vi "CANopenVM.vi"() -> ()   [LabVIEW 2020]
uses:
  <vilib>/Platform/TimedLoop/XDataNode/timing_clust.ctl
  <vilib>/Platform/TimedLoop/XDataNode/nitl_modes.ctl
  <vilib>/Platform/TimedLoop/XDataNode/wakeup.ctl
  <vilib>/CANopenLib/CANOPEN.llb/CANopen Interface Create.vi
  <vilib>/CANopenLib/CANOPEN.llb/CANopen SDO Create.vi
  <vilib>/CANopenLib/CANOPEN.llb/CANopen SDO Write [I16].vi
  <vilib>/CANopenLib/CANOPEN.llb/CANopen SDO Close.vi
  <vilib>/CANopenLib/CANOPEN.llb/CANopen SYNC Create.vi
  <vilib>/CANopenLib/CANOPEN.llb/CANopen RPDO Create.vi
  <vilib>/CANopenLib/CANOPEN.llb/CANopen TPDO Create.vi
  <vilib>/CANopenLib/CANOPEN.llb/CANopen SYNC Start.vi
  <vilib>/CANopenLib/CANOPEN.llb/CANopen RPDO Start.vi
  <vilib>/CANopenLib/CANOPEN.llb/CANopen TPDO Start.vi
  <vilib>/CANopenLib/CANOPEN.llb/CANopen Fetch from Data [I32].vi
  <vilib>/CANopenLib/CANOPEN.llb/CANopen SYNC Close.vi
  <vilib>/CANopenLib/CANOPEN.llb/CANopen RPDO Close.vi
  <vilib>/CANopenLib/CANOPEN.llb/CANopen TPDO Close.vi
  <vilib>/CANopenLib/CANOPEN.llb/CANopen Interface Close.vi
  <vilib>/Platform/TimedLoop/XDataNode/XDataNode.xnode
  <vilib>/Platform/TimedLoop/XDataNode/XDNodeRunTimeDep.lvlib
panel:
  in  "数值":i16
  in  "RPDO data":u8[](array[numeric])=[0, 0, 0, 0, 0, 0, 0, 0]
  out "实际速度":i32
  in  "Set Target Vilocity":i16
  in  "stop":bool
  out "timestamp":timestamp=timestamp(11705972400 s since 1904-01-01)
  out "channel data read":i32
  out "CANopen raw data read":u8[](array[numeric])
  in  "buffer size (0)":u16=10
  in  "TPDO channel read":u8(ring)=1 items=["PDO 1", "PDO 2", "PDO 3", "PDO 4"]
  in  "RPDO channel write":u8(ring)=1 items=["PDO 1", "PDO 2", "PDO 3", "PDO 4"]
  in  "period (ms)":i64=10
  out "completion code 2":u32
  out "completion code 1":u32
  in  "batch SDO name":string="NiMotion_VM"
  in  "node-ID":u8=1 min=1 max=127 step=1
  in  "baud rate":u32(ring) items=["1 Mbit/s"=0, "800 kbit/s"=1, "500 kbit/s"=2, "250 kbit/s"=3, "125 kbit/s"=4, "50 kbit/s"=6, "20 kbit/s"=7, "10 kbit/s"=8]
  in  "CANopen interface":u32(ring) items=["CANopen01", "CANopen02", "CANopen03", "CANopen04", "CANopen05", "CANopen06", "CANopen07", "CANopen08", "CANopen09", "CANopen10", "CANopen11", "CANopen12", "CANopen13", "CANopen14", "CANopen15", "CANopen16", "CANopen17", "CANopen18", "CANopen19", "CANopen20", "CANopen21", "CANopen22", "CANopen23", "CANopen24", "CANopen25", "CANopen26", "CANopen27", "CANopen28", "CANopen29", "CANopen30", "CANopen31", "CANopen32"]
  # "601 2B 02 20 01 00 00 00 00"
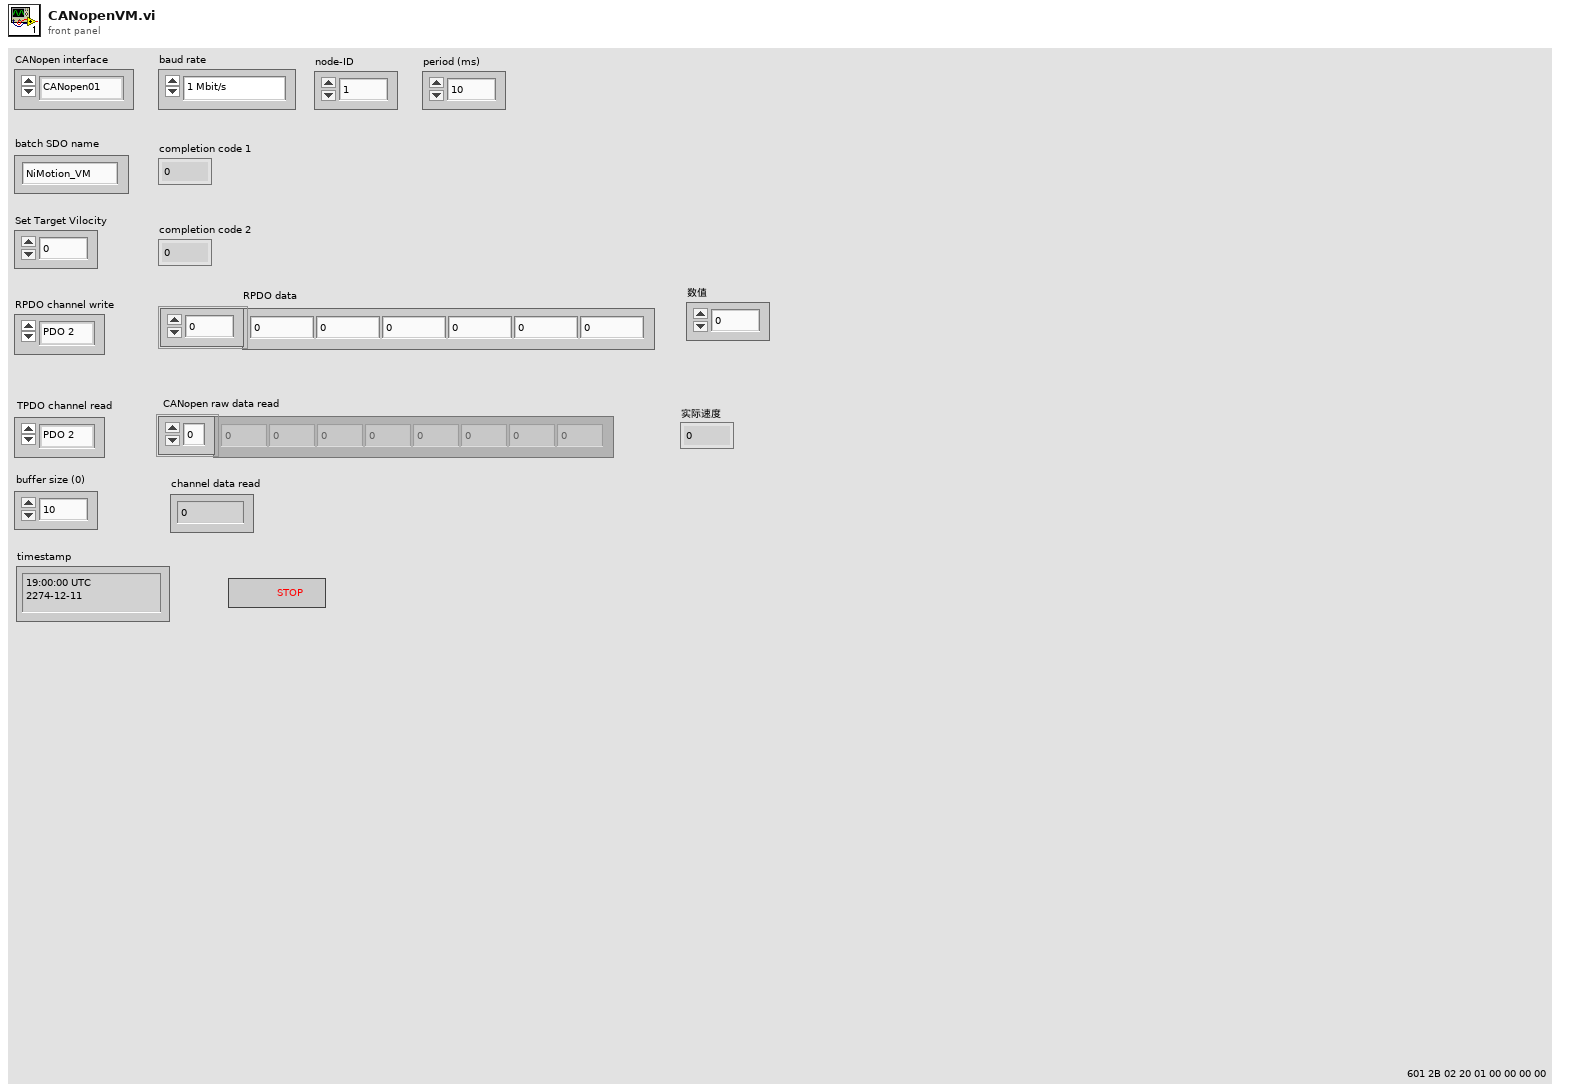
[diagram p1: front panel]
types:
  T1 = typedef "XDNodeRunTimeDep.lvlib/timing_clust.ctl" = cluster{"Expected End [f-1]":u64, "Actual End [f-1]":u64, "Finished Late? [f-1]":bool, "Expected End [i-1]":u64, "Actual End [i-1]":u64, "Finished Late? [i-1]":bool, "Expected Start [i]":u64, "Actual Start [i]":u64, "Expected Start [f]":u64, "Actual Start [f]":u64, "Source Name":string, "Structure Name":string, "Period":i64, "Deadline":i64, "Offset":i64, "Start":i64, "Priority":i32, "Timeout":i32, "Mode":T2, "Wakeup Reason":T3, "Error":errorcluster, "Source Type":string, "Secondary Source Type":string, "Global End Time":u64, "Global Start Time":u64, "Frame Duration":u64, "Iteration Duration":u64, "Assigned CPU":i32, "I/O Scan Engine Mode":u32}
  T2 = typedef "XDNodeRunTimeDep.lvlib/nitl_modes.ctl" = enum32{"No Change", "Process missed periods, maintain original phase", "Discard missed periods, maintain original phase", "Process missed periods, ignore original phase", "Discard missed periods, ignore original phase"}
  T3 = typedef "XDNodeRunTimeDep.lvlib/wakeup.ctl" = enum32{"Normal", "Aborted", "Asynchronous wakeup", "Timing source error", "Timed loop error", "Timeout"}
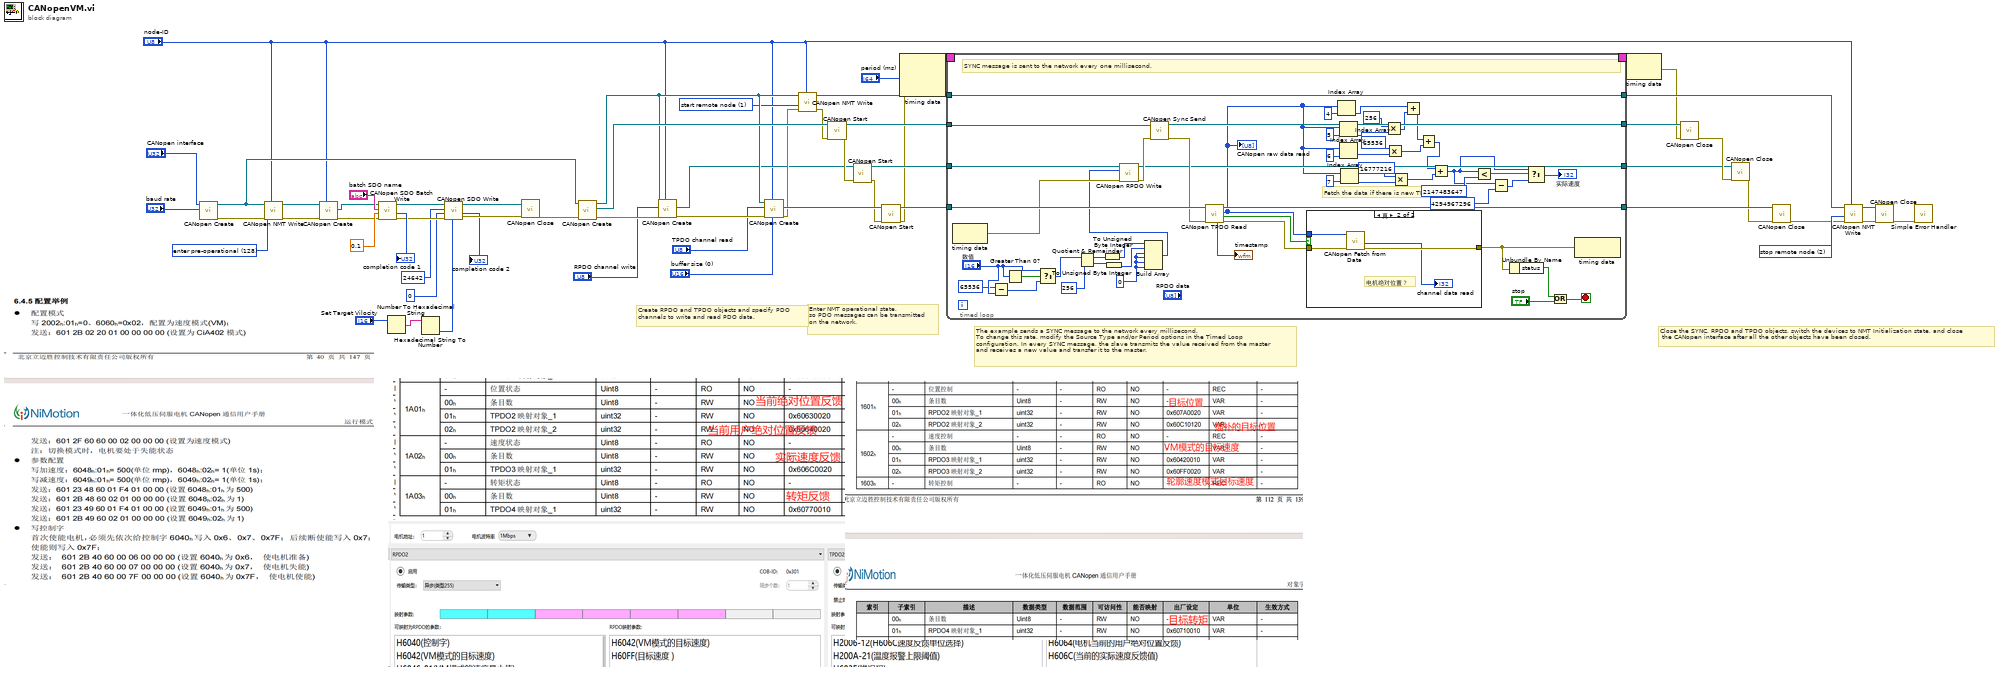
[diagram p0: block diagram]
diagram:
  w20 = u16 2 items=["start remote node"=1, "stop remote node"=2, "enter pre-operational"=128, "reset node"=129, "reset communication"=130] ("command")
  w35 = u16 1 items=["start remote node"=1, "stop remote node"=2, "enter pre-operational"=128, "reset node"=129, "reset communication"=130] ("command")
  w53 = u16 128 items=["start remote node"=1, "stop remote node"=2, "enter pre-operational"=128, "reset node"=129, "reset communication"=130] ("command")
  # "Close the SYNC, RPDO and TPDO objects, switch the devices to NMT Initialization state, and close\n the CANopen interface after all the other objects have been closed."
  # "The example sends a SYNC message to the network every millisecond.\nTo change this rate, modify the Source Type and/or Period options in the Timed Loop\nconfiguration. In every SYNC message, the slave transmits the value received from the master\nand receives a new value and transfer it to the master."
  # "Enter NMT operational state,\nso PDO messages can be transmitted\non the network."
  # "Create RPDO and TPDO objects and specify PDO \nchannels to write and read PDO data."
  n1 = call-poly <vilib>:"CANopen Create.vi"("baud rate"="baud rate", "interface name"="CANopen interface") -> ("error out"=w54:errorcluster, "interface object out"=w26:refnum<k20>)  [unwired: 8 in]
  n2 = call <vilib>:"CANopen NMT Write.vi"("node-ID (0)"="node-ID", "error in (no error)"=w54, "command"=w53, "interface object in"=w26) -> ("error out"=w57:errorcluster, "interface object out"=w58:refnum<k20>)  [unwired: 6 in]
  n3 = call-poly <vilib>:"CANopen Create.vi"("node-ID"="node-ID", "error in (no error)"=w57, "interface object in"=w58) -> ("error out"=w44:errorcluster, "SDO object out"=w50:refnum<k20>)  [unwired: 6 in, 1 out]
  n4 = call <vilib>:"CANopen SDO Batch Write.vi"("error in (no error)"=w44, "timeout (1s)"=0.1 ("timeout (0s)"), "batch SDO name"="batch SDO name", "SDO object in"=w50) -> ("error out"=w45:errorcluster, "completion code"=→"completion code 1":u32, "SDO object out"=w48:refnum<k20>)  [unwired: 5 in]
  n5 = Number To Hexadecimal String(2:"Set Target Vilocity") -> (0:w3:string)  [unwired: 1 in]
  n6 = Hexadecimal String To Number(string=w3) -> (number=w1:u32)  [unwired: 2 in, 1 out]
  n7 = call-poly <vilib>:"CANopen SDO Write.vi"("I16 data"=w1, "error in (no error)"=w45, "object sub-index (0)"=u8 0, "object index"=u16 24642, "SDO object in"=w48) -> ("error out"=w46:errorcluster, "completion code"=→"completion code 2":u32, "SDO object out"=w47:refnum<k20>)  [unwired: 4 in]
  n8 = call-poly <vilib>:"CANopen Close.vi"("error in (no error)"=w46, "SDO object in"=w47) -> ("error out"=w25:errorcluster)  [unwired: 9 in]
  n9 = call-poly <vilib>:"CANopen Create.vi"("error in (no error)"=w25, "interface object in"=w26) -> ("error out"=w38:errorcluster, "SYNC object out"=w37:refnum<k20>, "interface object out"=w36:refnum<k20>)  [unwired: 7 in]
  n10 = call-poly <vilib>:"CANopen Create.vi"("node-ID"="node-ID", "error in (no error)"=w38, "PDO channel"="RPDO channel write", "interface object in"=w36) -> ("error out"=w30:errorcluster, "RPDO object out"=w29:refnum<k20>)  [unwired: 5 in, 1 out]
  n11 = call-poly <vilib>:"CANopen Create.vi"("buffer size (0)"="buffer size (0)", "node-ID"="node-ID", "error in (no error)"=w30, "PDO channel"="TPDO channel read", "interface object in"=w36) -> ("error out"=w34:errorcluster, "TPDO object out"=w40:refnum<k20>)  [unwired: 4 in, 1 out]
  n12 = call <vilib>:"CANopen NMT Write.vi"("node-ID (0)"="node-ID", "error in (no error)"=w34, "command"=w35, "interface object in"=w36) -> ("error out"=w33:errorcluster, "interface object out"=w9:refnum<k20>)  [unwired: 6 in]
  n13 = call-poly <vilib>:"CANopen Start.vi"("error in (no error)"=w33, "SYNC object in"=w37) -> ("error out"=w32:errorcluster, "SYNC object out"=w8:refnum<k20>)  [unwired: 8 in]
  n14 = call-poly <vilib>:"CANopen Start.vi"("error in (no error)"=w32, "RPDO object in"=w29) -> ("error out"=w31:errorcluster, "RPDO object out"=w7:refnum<k20>)  [unwired: 8 in]
  n15 = call-poly <vilib>:"CANopen Start.vi"("error in (no error)"=w31, "TPDO object in"=w40) -> ("error out"=w4:errorcluster, "TPDO object out"=w6:refnum<k20>)  [unwired: 8 in]
  n16 = node-c288("period (ms)", w4) -> (w24:T1)  [unwired: 1 in]
  n17 = timed-loop {
    timing: w24 -> [_]
    timing-out: [_] -> w23
    tunnel: w8 -> [w110]
    tunnel: [w97] -> w13
    tunnel: [w109] -> w19
    tunnel: w9 -> [w109]
    tunnel: w7 -> [w102]
    tunnel: w6 -> [w103]
    tunnel: [w99] -> w16
    tunnel: [w98] -> w17
    stop <- w108 stop-if-true
    w70 = u8 0 ("元素")
    # "Fetch the data if there is new TPDO."
    # "SYNC message is sent to the network every one millisecond."
    n18 = node-c288() -> (w77:errorcluster)  [unwired: 1 in]
    n19 = Subtract(x=u32 65536, y="数值") -> (x-y=w66:u32)
    n20 = Greater Than 0?(x="数值") -> (x > 0?=w67:bool)
    n21 = Select(t="数值", s=w67, f=w66) -> (s? t:f=w65:u32)
    n22 = Quotient & Remainder(x=w65, y=i16 256) -> (x-y*floor(x/y)=w75:u32, floor(x/y)=w73:u32)
    n23 = To Unsigned Byte Integer(number=w75) -> (unsigned 8bit integer=w74:u8)
    n24 = To Unsigned Byte Integer(number=w73) -> (unsigned 8bit integer=w72:u8)
    n25 = Build Array(w74, w72, w70, w70, w70, w70) -> (w71:u8[])
    n26 = call <vilib>:"CANopen RPDO Write.vi"("error in (no error)"=w77, "data"=w71, "RPDO object in"=w102) -> ("error out"=w101:errorcluster, "RPDO object out"=w98:refnum<k20>)  [unwired: 7 in]
    n27 = call <vilib>:"CANopen Sync Send.vi"("error in (no error)"=w101, "SYNC object in"=w110) -> ("error out"=w100:errorcluster, "SYNC object out"=w97:refnum<k20>)  [unwired: 8 in]
    n28 = call <vilib>:"CANopen TPDO Read.vi"("error in (no error)"=w100, "TPDO object in"=w103) -> ("error out"=w104:errorcluster, "new data?"=w96:bool, "data"=w91:u8[], "TPDO object out"=w99:refnum<k20>, "timestamp"=→"timestamp":timestamp)  [unwired: 5 in]
    "CANopen raw data read" <- w91
    n29 = case shown="真" w96 {
      tunnel: w104 -> [w116 w120]
      tunnel: w91 -> [_ w119]
      tunnel: [w116 w118] -> w95
      frame False {
      }
      frame True {
        # "电机绝对位置？"
        n30 = call-poly <vilib>:"CANopen Fetch from Data.vi"("error in (no error)"=w120, "CANopen data in"=w119) -> ("error out"=w118:errorcluster, "signed 32-bit integer"=→"channel data read":i32)  [unwired: 7 in, 1 out]
      }
    }
    n31 = Index Array(array=w91, index=4 ("索引")) -> (element=w82:u8)
    n32 = Index Array(array=w91, index=5 ("索引")) -> (element=w89:u8)
    n33 = Index Array(array=w91, index=6 ("索引")) -> (element=w87:u8)
    n34 = Index Array(array=w91, index=7 ("索引")) -> (element=w85:u8)
    n35 = Multiply(x=u32 256, y=w89) -> (x*y=w83:u32)
    n36 = Multiply(x=u32 65536, y=w87) -> (x*y=w80:u32)
    n37 = Multiply(x=u32 16777216, y=w85) -> (x*y=w78:u32)
    n38 = Add(x=w82, y=w83) -> (x+y=w81:u32)
    n39 = Add(x=w81, y=w80) -> (x+y=w79:u32)
    n40 = Add(x=w79, y=w78) -> (x+y=w62:u32)
    n41 = Less?(x=w62, y=u64 2147483647) -> (x < y?=w63:bool)
    n42 = Subtract(x=w62, y=u64 4294967296) -> (x-y=w60:u64)
    n43 = Unbundle By Name(w95) -> ("status"=w106:bool)
    n44 = Select(t=w62, s=w63, f=w60) -> (s? t:f=→"实际速度":u64)
    n45 = Or(x=w106, y="stop") -> (x .or. y?=w108:bool)
    n46 = node-c288(w95) -> ()  [unwired: 1 out]
  }
  n47 = node-c288(w23) -> (w11:errorcluster)
  n48 = call-poly <vilib>:"CANopen Close.vi"("error in (no error)"=w11, "SYNC object in"=w13) -> ("error out"=w18:errorcluster)  [unwired: 9 in]
  n49 = call-poly <vilib>:"CANopen Close.vi"("error in (no error)"=w18, "RPDO object in"=w17) -> ("error out"=w15:errorcluster)  [unwired: 9 in]
  n50 = call-poly <vilib>:"CANopen Close.vi"("error in (no error)"=w15, "TPDO object in"=w16) -> ("error out"=w14:errorcluster)  [unwired: 9 in]
  n51 = call <vilib>:"CANopen NMT Write.vi"("node-ID (0)"="node-ID", "error in (no error)"=w14, "command"=w20, "interface object in"=w19) -> ("error out"=w22:errorcluster, "interface object out"=w21:refnum<k20>)  [unwired: 6 in]
  n52 = call-poly <vilib>:"CANopen Close.vi"("error in (no error)"=w22, "interface object in"=w21) -> ("error out"=w12:errorcluster)  [unwired: 9 in]
  n53 = call <vilib>:"Simple Error Handler.vi"("error in (no error)"=w12) -> ()  [unwired: 4 in, 5 out]
